vi "Destroy Request Events.vi"(8 "error in":errorcluster) -> (0 "error out":errorcluster)   [LabVIEW 2020, in "G-AI Core.lvlib"]
doc: "Destroy the requests user events, even if there is an incoming error.\n\n<b>NOTE</b>: The contents of this VI are automatically generated and modified by the <b>Tools > DQMH Consortium > DQMH</b> utilities. Consider using those utilities instead of making your own modifications to this VI.\n_____\nBased on DQMH Dev Tools: Project Template 7.1.2.1547."
uses:
  G-AI Core.lvlib
panel:
  # "NOTE: The contents of this VI are automatically generated and modified by the Tools > DQMH Consortium > DQMH utilities. Consider using those utilities instead of making your own modifications to this VI."
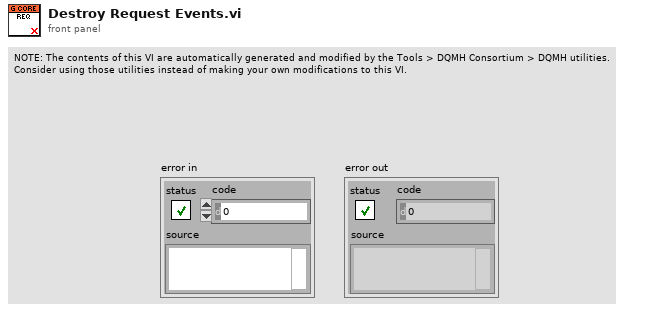
[diagram p1: front panel]
types:
  T1 = typedef "G-AI Core.lvlib/Request Events--cluster.ctl" = cluster{"Stop Module":refnum<user-event>, "Show Panel":refnum<user-event>, "Hide Panel":refnum<user-event>, "Get Module Execution Status":refnum<user-event>, "Show Diagram":refnum<user-event>, "Store Reference":refnum<user-event>, "Get Reference":refnum<user-event>, "New VI":refnum<user-event>, "Open VI Reference":refnum<user-event>}
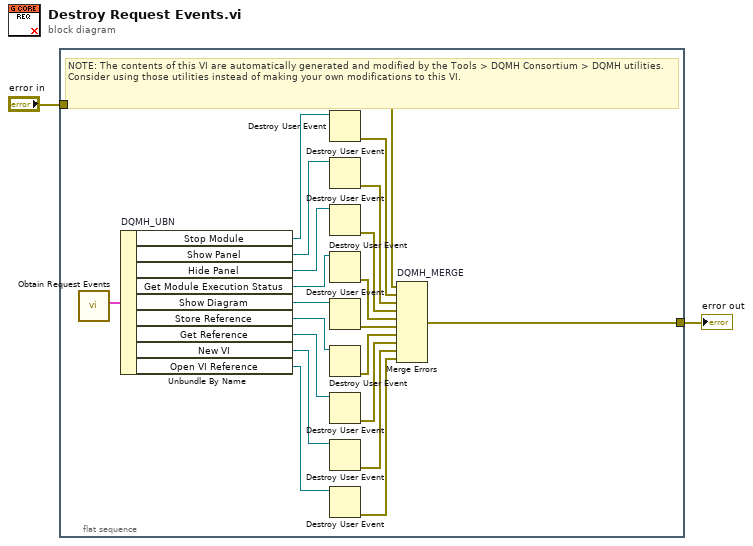
[diagram p0: block diagram]
diagram:
  n1 = flat-sequence {
    tunnel: [w22] -> w2
    tunnel: "error in" -> [w15]
    frame #0 {
      # "NOTE: The contents of this VI are automatically generated and modified by the Tools > DQMH Consortium > DQMH utilities. Consider using those utilities instead of making your own modifications to this VI."
      n2 = call "Obtain Request Events.vi"() -> ("G-AI Core Request Events"=w21:T1)  [unwired: 10 in, 1 out]
      n3 = Unbundle By Name "DQMH_UBN"(w21) -> ("Stop Module"=w20:refnum<user-event>, "Show Panel"=w17:refnum<user-event>, "Hide Panel"=w16:refnum<user-event>, "Get Module Execution Status"=w13:refnum<user-event>, "Show Diagram"=w11:refnum<user-event>, "Store Reference"=w9:refnum<user-event>, "Get Reference"=w7:refnum<user-event>, "New VI"=w5:refnum<user-event>, "Open VI Reference"=w3:refnum<user-event>)
      n4 = Destroy User Event(user event=w20) -> (error out=w23:errorcluster)  [unwired: 1 in]
      n5 = Destroy User Event(user event=w17) -> (error out=w19:errorcluster)  [unwired: 1 in]
      n6 = Destroy User Event(user event=w16) -> (error out=w18:errorcluster)  [unwired: 1 in]
      n7 = Destroy User Event(user event=w13) -> (error out=w14:errorcluster)  [unwired: 1 in]
      n8 = Destroy User Event(user event=w11) -> (error out=w12:errorcluster)  [unwired: 1 in]
      n9 = Destroy User Event(user event=w9) -> (error out=w10:errorcluster)  [unwired: 1 in]
      n10 = Destroy User Event(user event=w7) -> (error out=w8:errorcluster)  [unwired: 1 in]
      n11 = Destroy User Event(user event=w5) -> (error out=w6:errorcluster)  [unwired: 1 in]
      n12 = Destroy User Event(user event=w3) -> (error out=w4:errorcluster)  [unwired: 1 in]
      n13 = Merge Errors "DQMH_MERGE"(w15, w23, w19, w18, w14, w12, w10, w8, w6, w4) -> (w22:errorcluster)
    }
  }
  "error out" <- w2
